vi "Edit Substeps PWM Input.vi"(8 "error in":errorcluster, 10 "PWM Input In":T1, 11 "Sequence Context In":refnum<k7>) -> (0 "error out":errorcluster, 2 "PWM Input Out":T1, 3 "Report Text":string)   [LabVIEW 2023, in "LTT_TeststandSteptypes.lvlib"]
doc: "This VI Analog Input Signal Map and Multinumberic Edit Sub step"
uses:
  LTT_TeststandSteptypes.lvlib
  HardwareAbstractionLayer_LVOOP/PWM Input/NI PWM Input_class/NI PWM DAQ/Control/PWMInputEdit.ctl
  HardwareAbstractionLayer_LVOOP/Database/SQL Public VI/Control/DB Options.ctl
  <vilib>/addons/TestStand/_TSUtility.llb/TestStand - Start Modal Dialog (Sequence Context).vi
  <vilib>/addons/TestStand/_TSUtility.llb/TestStand - End Modal Dialog (Sequence Context).vi
  HardwareAbstractionLayer_LVOOP/Database/Database.lvclass
  HardwareAbstractionLayer_LVOOP/PWM Input/NI PWM Input_class/NI PWM Input.lvclass
panel:
  in  "Close":bool
  in  "OK":bool
  in  "Station No":i32
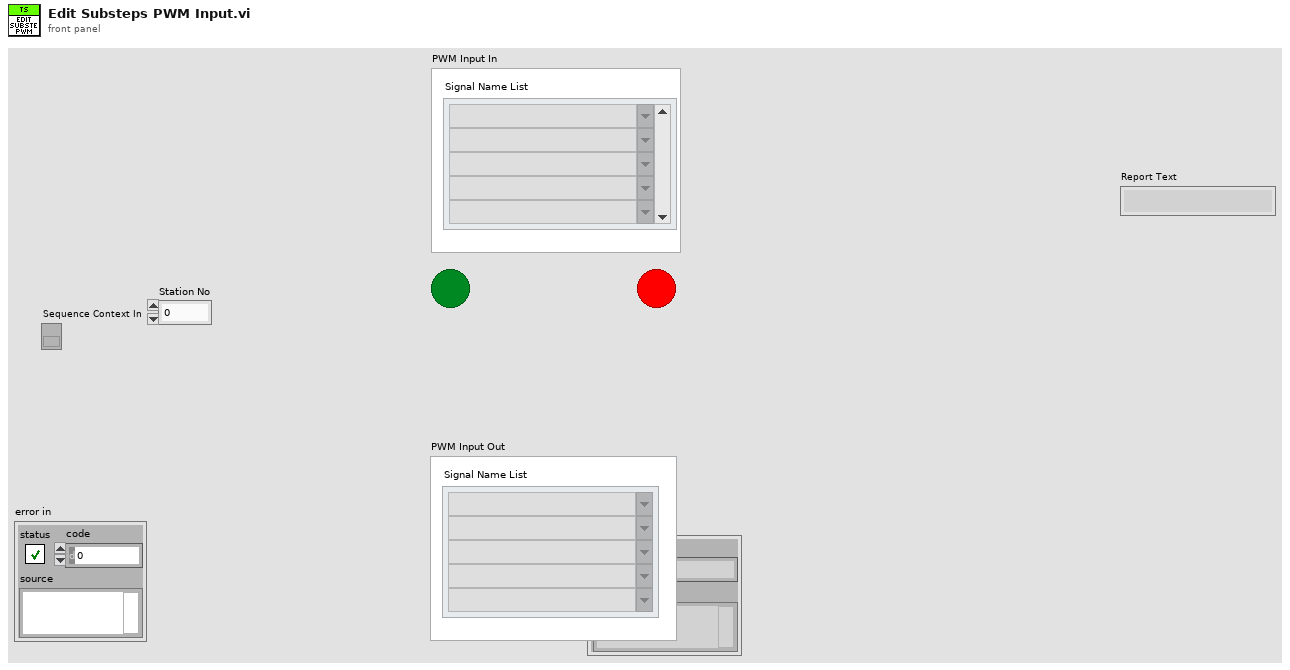
[diagram p1: front panel]
types:
  T1 = typedef "HardwareAbstractionLayer_LVOOP.lvlib/NI PWM Input.lvclass/PWMInputEdit.ctl" = cluster{"Signal Name List":string[]}
  T2 = typedef "HardwareAbstractionLayer_LVOOP.lvlib/Database.lvclass/DB Options.ctl" = enum16{"Init", "Select Data", "Insert Data", "Update Data", "Delete Data", "Execute Query", "Create Schema", "Create Table", "List Tables", "List Columns", "Close"}
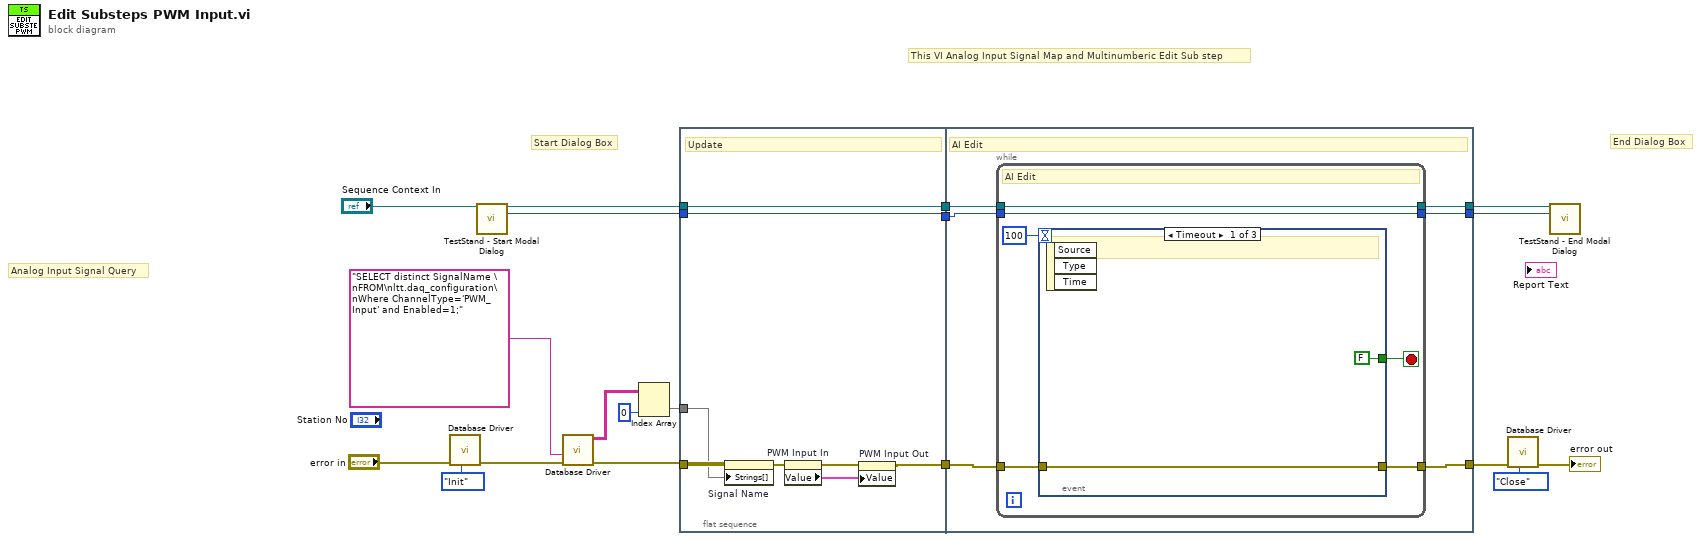
[diagram p0: block diagram]
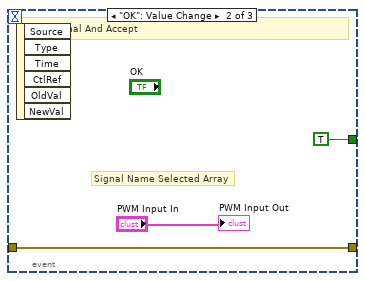
[diagram p2: hidden frame]
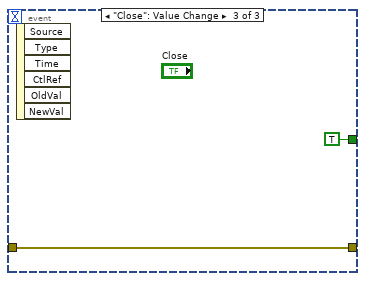
[diagram p3: hidden frame]
diagram:
  # "Analog Input Signal Query"
  # "This VI Analog Input Signal Map and Multinumberic Edit Sub step"
  # "End Dialog Box"
  # "Start Dialog Box"
  n1 = call "Database Driver.vi"("Options"=DB_Options."Init", "error in"="error in") -> ("error out"=w5:errorcluster)  [unwired: 6 in, 3 out]
  n2 = call-poly <vilib>:"TestStand - Start Modal Dialog.vi"("Sequence Context In"="Sequence Context In") -> ("Sequence Context Out"=w16:refnum<k7>, "Modal ID"=w15:i32)  [unwired: 10 in, 3 out]
  n3 = call "Database Driver.vi"("error in"=w5, "SQL query"="SELECT distinct SignalName \nFROM\nltt.daq_configuration\nWhere ChannelType='PWM_Input' and Enabled=1;") -> ("error out"=w7:errorcluster, "data"=w10:string[][])  [unwired: 6 in, 2 out]
  n4 = Index Array(array=w10, index (col)=0 ("disabled index (col)")) -> (element=w8:string[])  [unwired: 1 in]
  n5 = flat-sequence {
    tunnel: w7 -> [w23]
    tunnel: [w20] -> w19
    tunnel: w8 -> [w24]
    tunnel: w16 -> [w27]
    tunnel: w15 -> [w26]
    tunnel: [w27] -> w14
    tunnel: [w26] -> w13
    tunnel: w19 -> [w33]
    tunnel: [w32] -> w18
    tunnel: w14 -> [w31]
    tunnel: [w30] -> w12
    tunnel: w13 -> [w29]
    tunnel: [w28] -> w11
    frame #0 {
      # "Update"
      n6 = property on="Signal Name" class="CmbBox"(error in=w23, "Strings[]"=w24) -> (error out=w22:errorcluster)  [unwired: 1 in, 1 out]
      n7 = property on="PWM Input In" class="Clust (strict)"(error in=w22) -> (error out=w21:errorcluster, "Value"=w25:T1)  [unwired: 1 in, 1 out]
      n8 = property on="PWM Input Out" class="Clust (strict)"(error in=w21, "Value"=w25) -> (error out=w20:errorcluster)  [unwired: 1 in, 1 out]
    }
    frame #1 {
      # "AI Edit"
      n9 = while {
        tunnel: w33 -> [w36]
        tunnel: [w35] -> w32
        tunnel: w31 -> [w39]
        tunnel: [w39] -> w30
        tunnel: w29 -> [w38]
        tunnel: [w38] -> w28
        stop <- w34 stop-if-true
        # "AI Edit"
        n10 = event shown="[0] Timeout" {
          selector: _ -> [_ _ _]
          dyn-events: _ -> [_ _ _]
          timeout: 100 -> [_ _ _]
          tunnel: w36 -> [w41 w44 w45]
          tunnel: [w41 w44 w45] -> w35
          tunnel: [FALSE TRUE TRUE] -> w34
          event Timeout {
            # "TimeOut"
            n11 = event-data() -> ()  [unwired: 1 in, 3 out]
          }
          event "OK": Value Change {
            # "Signal Name Selected Array"
            # "Select Signal And Accept"
            n12 = event-data() -> ()  [unwired: 1 in, 6 out]
            "PWM Input Out" <- "PWM Input In"
          }
          event "Close": Value Change {
            n13 = event-data() -> ()  [unwired: 1 in, 6 out]
          }
        }
      }
    }
  }
  n14 = call "Database Driver.vi"("Options"=DB_Options."Close", "error in"=w18) -> ("error out"=→"error out":errorcluster)  [unwired: 6 in, 3 out]
  n15 = call-poly <vilib>:"TestStand - End Modal Dialog.vi"("Sequence Context In"=w12, "Modal ID"=w11) -> ()  [unwired: 13 in, 1 out]
